vi "inches to ticks.vi"(10 "x":dbl) -> (2 "x*y":dbl)   [LabVIEW 2016]
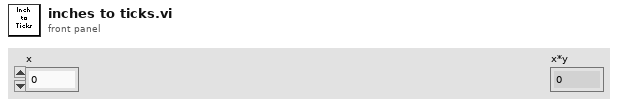
[diagram p1: front panel]
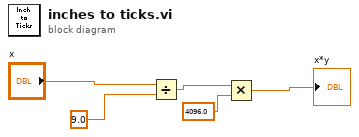
[diagram p0: block diagram]
diagram:
  n1 = Divide(x="x", y=9.0) -> (x/y=w3:dbl)
  n2 = Multiply(x=w3, y=4096.0) -> (x*y=→"x*y":dbl)
